vi "CalcMinDist.vi"(4 "PointY":dbl(slide) scale=-3.0..3.0, 6 "PointX":dbl(slide) scale=-3.0..3.0, 7 "Angle":dbl=35.0, 8 "Line2Y":dbl=4.0, 9 "Line2X":dbl=2.0, 10 "Line1Y":dbl format="%#_13g", 11 "Line1X":dbl format="%#_13g") -> (0 "In Angle?":bool, 3 "Result":dbl)   [LabVIEW 2014]
uses:
  <vilib>/express/express arith-compare/Formula/XNode/ExpressFormulaBlockNode.xnode
panel:
  in  "milliseconds to wait":u32
  out "XY Graph":cluster{dbl[], dbl[]}[](graph)
  in  "cluster":T1
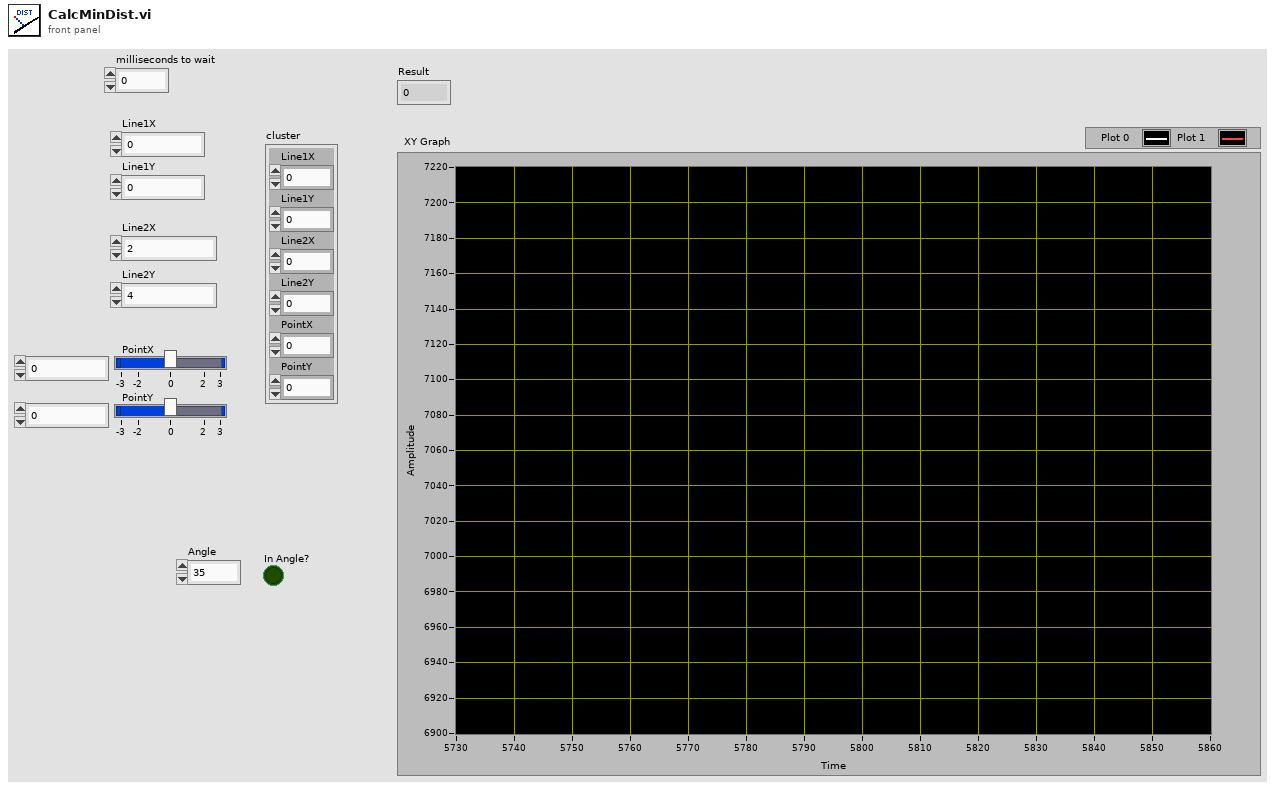
[diagram p1: front panel]
types:
  T1 = cluster{"Line1X":dbl, "Line1Y":dbl, "Line2X":dbl, "Line2Y":dbl, "PointX":dbl, "PointY":dbl}
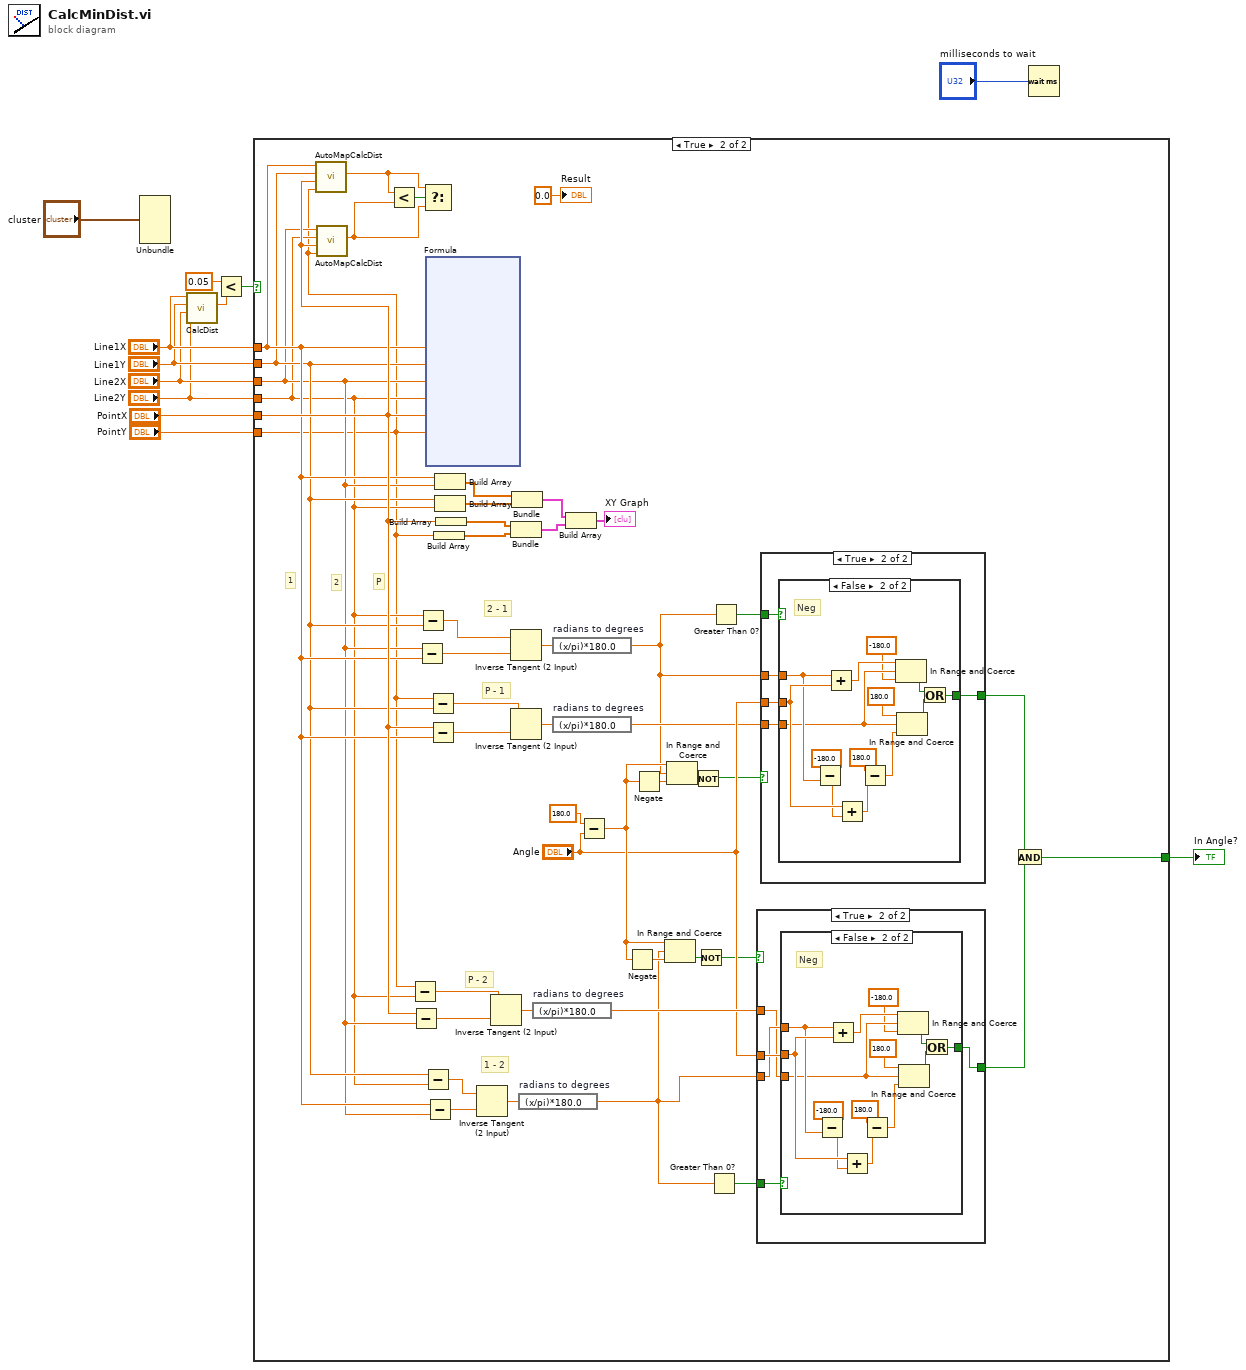
[diagram p0: block diagram]
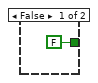
[diagram p2: hidden frame]
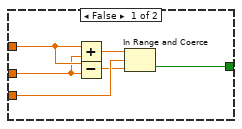
[diagram p3: hidden frame]
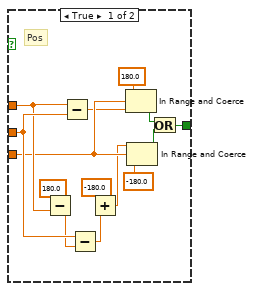
[diagram p4: hidden frame]
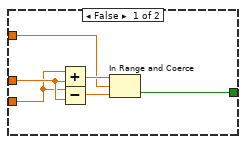
[diagram p5: hidden frame]
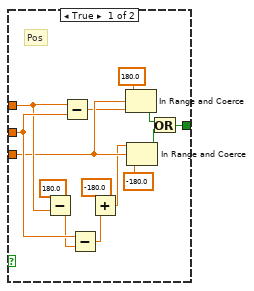
[diagram p6: hidden frame]
diagram:
  n1 = Unbundle("cluster") -> ()  [unwired: 6 out]
  n2 = call "CalcDist.vi"("Y2"="Line2Y", "X2"="Line2X", "Y1"="Line1Y", "X1"="Line1X") -> ("Distance"=w8:dbl)  [unwired: 7 in]
  n3 = Less?(x=0.05, y=w8) -> (x < y?=w1:bool)
  n4 = case shown="True" w1 {
    tunnel: "PointY" -> [_ w15]
    tunnel: "PointX" -> [_ w38]
    tunnel: "Line1X" -> [_ w20]
    tunnel: "Line1Y" -> [_ w19]
    tunnel: "Line2X" -> [_ w18]
    tunnel: "Line2Y" -> [_ w17]
    tunnel: [FALSE w16] -> w2
    frame False {
    }
    frame True {
      # "P"
      # "2"
      # "1"
      # "1 - 2"
      # "P - 2"
      # "2 - 1"
      # "P - 1"
      n5 = call "AutoMapCalcDist.vi"("Y2"=w15, "X2"=w38, "Y1"=w19, "X1"=w20) -> ("Distance"=w40:dbl)  [unwired: 7 in]
      n6 = call "AutoMapCalcDist.vi"("Y2"=w15, "X2"=w38, "Y1"=w17, "X1"=w18) -> ("Distance"=w39:dbl)  [unwired: 7 in]
      n7 = Less?(x=w40, y=w39) -> (x < y?=w41:bool)
      n8 = Subtract(x=w15, y=w17) -> (x-y=w45:dbl)
      n9 = Subtract(x=w38, y=w18) -> (x-y=w46:dbl)
      n10 = Subtract(x=w18, y=w20) -> (x-y=w51:dbl)
      n11 = Subtract(x=w17, y=w19) -> (x-y=w50:dbl)
      n12 = Select(t=w40, s=w41, f=w39) -> ()  [unwired: 1 out]
      n13 = Subtract(x=w19, y=w17) -> (x-y=w44:dbl)
      n14 = Subtract(x=w20, y=w18) -> (x-y=w43:dbl)
      n15 = xnode "Formula"("x1"=w20, "y1"=w19, "x2"=w18, "y2"=w17, "xc"=w38, "yc"=w15) -> ()  [unwired: 1 in, 2 out]
      n16 = Subtract(x=w15, y=w19) -> (x-y=w47:dbl)
      n17 = Subtract(x=w38, y=w20) -> (x-y=w48:dbl)
      n18 = Build Array(w15) -> (w57:dbl[])
      n19 = Build Array(w20, w18) -> (w60:dbl[])
      n20 = Build Array(w19, w17) -> (w59:dbl[])
      n21 = Build Array(w38) -> (w58:dbl[])
      n22 = Inverse Tangent (2 Input)(1:w43, 2:w44) -> (0:w42:dbl)
      n23 = Inverse Tangent (2 Input)(1:w46, 2:w45) -> (0:w49:dbl)
      n24 = Bundle(w58, w57) -> (w56:cluster{dbl[], dbl[]})  [unwired: 1 in]
      n25 = Inverse Tangent (2 Input)(1:w51, 2:w50) -> (0:w53:dbl)
      n26 = Inverse Tangent (2 Input)(1:w48, 2:w47) -> (0:w52:dbl)
      n27 = Bundle(w60, w59) -> (w55:cluster{dbl[], dbl[]})  [unwired: 1 in]
      n28 = expression code="(x/pi)*180.0" "radians to degrees"(w42) -> (w22:dbl)
      n29 = expression code="(x/pi)*180.0" "radians to degrees"(w49) -> (w31:dbl)
      n30 = expression code="(x/pi)*180.0" "radians to degrees"(w53) -> (w23:dbl)
      n31 = expression code="(x/pi)*180.0" "radians to degrees"(w52) -> (w25:dbl)
      n32 = Build Array(w55, w56) -> (→"XY Graph":cluster{dbl[], dbl[]}[])
      n33 = Subtract(x=180.0, y="Angle") -> (x-y=w32:dbl)
      n34 = Negate(x=w32) -> (-x=w33:dbl)
      n35 = Negate(x=w32) -> (-x=w34:dbl)
      n36 = In Range and Coerce(upper limit=w32, x=w22, lower limit=w33) -> (In Range?=w29:bool)  [unwired: 1 out]
      n37 = In Range and Coerce(upper limit=w32, x=w23, lower limit=w34) -> (In Range?=w30:bool)  [unwired: 1 out]
      n38 = Not(x=w30) -> (.not. x?=w26:bool)
      n39 = Not(x=w29) -> (.not. x?=w27:bool)
      n40 = Greater Than 0?(x=w22) -> (x > 0?=w21:bool)
      n41 = Greater Than 0?(x=w23) -> (x > 0?=w24:bool)
      n42 = case shown="True" w27 {
        tunnel: [w103 w106] -> w36
        tunnel: w31 -> [w102 w107]
        tunnel: "Angle" -> [w101 w109]
        tunnel: w22 -> [w100 w108]
        tunnel: w21 -> [_ w110]
        frame False {
          n43 = Add(x=w100, y=w101) -> (x+y=w105:dbl)
          n44 = Subtract(x=w100, y=w101) -> (x-y=w104:dbl)
          n45 = In Range and Coerce(upper limit=w105, x=w102, lower limit=w104) -> (In Range?=w103:bool)  [unwired: 1 out]
        }
        frame True {
          n46 = case shown="False" w110 {
            tunnel: [w119 w133] -> w106
            tunnel: w109 -> [w123 w137]
            tunnel: w107 -> [w115 w129]
            tunnel: w108 -> [w116 w130]
            frame True {
              # "Pos"
              n47 = Subtract(x=180.0, y=w116) -> (x-y=w122:dbl)
              n48 = Subtract(x=w116, y=w123) -> (x-y=w114:dbl)
              n49 = Subtract(x=w123, y=w122) -> (x-y=w120:dbl)
              n50 = Add(x=-180.0, y=w120) -> (x+y=w112:dbl)
              n51 = In Range and Coerce(upper limit=180.0, x=w115, lower limit=w114) -> (In Range?=w117:bool)  [unwired: 1 out]
              n52 = In Range and Coerce(upper limit=w112, x=w115, lower limit=-180.0) -> (In Range?=w118:bool)  [unwired: 1 out]
              n53 = Or(x=w117, y=w118) -> (x .or. y?=w119:bool)
            }
            frame False {
              # "Neg"
              n54 = Subtract(x=-180.0, y=w130) -> (x-y=w136:dbl)
              n55 = Add(x=w130, y=w137) -> (x+y=w128:dbl)
              n56 = Add(x=w137, y=w136) -> (x+y=w134:dbl)
              n57 = Subtract(x=180.0, y=w134) -> (x-y=w126:dbl)
              n58 = In Range and Coerce(upper limit=w128, x=w129, lower limit=-180.0) -> (In Range?=w131:bool)  [unwired: 1 out]
              n59 = In Range and Coerce(upper limit=180.0, x=w129, lower limit=w126) -> (In Range?=w132:bool)  [unwired: 1 out]
              n60 = Or(x=w131, y=w132) -> (x .or. y?=w133:bool)
            }
          }
        }
      }
      n61 = case shown="True" w26 {
        tunnel: w25 -> [w66 w68]
        tunnel: [w63 w70] -> w37
        tunnel: w23 -> [w62 w67]
        tunnel: "Angle" -> [w61 w69]
        tunnel: w24 -> [_ w71]
        frame False {
          n62 = Add(x=w62, y=w61) -> (x+y=w65:dbl)
          n63 = Subtract(x=w62, y=w61) -> (x-y=w64:dbl)
          n64 = In Range and Coerce(upper limit=w65, x=w66, lower limit=w64) -> (In Range?=w63:bool)  [unwired: 1 out]
        }
        frame True {
          n65 = case shown="False" w71 {
            tunnel: [w80 w94] -> w70
            tunnel: w69 -> [w84 w98]
            tunnel: w68 -> [w76 w90]
            tunnel: w67 -> [w77 w91]
            frame True {
              # "Pos"
              n66 = Subtract(x=180.0, y=w77) -> (x-y=w83:dbl)
              n67 = Subtract(x=w77, y=w84) -> (x-y=w75:dbl)
              n68 = Subtract(x=w84, y=w83) -> (x-y=w81:dbl)
              n69 = Add(x=-180.0, y=w81) -> (x+y=w73:dbl)
              n70 = In Range and Coerce(upper limit=180.0, x=w76, lower limit=w75) -> (In Range?=w78:bool)  [unwired: 1 out]
              n71 = In Range and Coerce(upper limit=w73, x=w76, lower limit=-180.0) -> (In Range?=w79:bool)  [unwired: 1 out]
              n72 = Or(x=w78, y=w79) -> (x .or. y?=w80:bool)
            }
            frame False {
              # "Neg"
              n73 = Subtract(x=-180.0, y=w91) -> (x-y=w97:dbl)
              n74 = Add(x=w91, y=w98) -> (x+y=w89:dbl)
              n75 = Add(x=w98, y=w97) -> (x+y=w95:dbl)
              n76 = Subtract(x=180.0, y=w95) -> (x-y=w87:dbl)
              n77 = In Range and Coerce(upper limit=w89, x=w90, lower limit=-180.0) -> (In Range?=w92:bool)  [unwired: 1 out]
              n78 = In Range and Coerce(upper limit=180.0, x=w90, lower limit=w87) -> (In Range?=w93:bool)  [unwired: 1 out]
              n79 = Or(x=w92, y=w93) -> (x .or. y?=w94:bool)
            }
          }
        }
      }
      n80 = And(x=w37, y=w36) -> (x .and. y?=w16:bool)
      "Result" <- 0.0 ("Result")
    }
  }
  "In Angle?" <- w2
  n81 = Wait (ms)(milliseconds to wait="milliseconds to wait") -> ()  [unwired: 1 out]
